vi "Send Write Load Control.vi"(7 "Message Priority (Normal)":T3=enum."Normal", 8 "error in (no error)":errorcluster, 10 "Load_Control":T1, 11 "Message Enqueuer":refnum<class "Message Enqueuer.lvclass">) -> (0 "error out":errorcluster, 3 "Message Enqueuer out":refnum<class "Message Enqueuer.lvclass">)   [LabVIEW 2018, in "Load Actor.lvlib" / "Write Load Control Msg.lvclass"]
doc: "This VI sends the message to an actor."
uses:
  Write Load Control Msg.lvclass
  <vilib>/ActorFramework/Message Enqueuer/Message Enqueuer.lvclass
  <vilib>/ActorFramework/Message Enqueuer/Message Priority.ctl
  <vilib>/ORNL/CSEISMIC DDS/CSEISMIC DDS Base/Data Types/Load_Control.ctl
  <vilib>/ORNL/CSEISMIC DDS/CSEISMIC DDS Base/Data Types/Controls/DeviceID.ctl
  C:/Program Files (x86)/National Instruments/LabVIEW 2018/vi.lib/ActorFramework/Message/Message.lvclass
  Write Load Control Msg.lvclass/Write Load Control Msg.ctl
  <vilib>/ActorFramework/Message Enqueuer/Message Enqueuer.lvclass/Message Enqueuer.ctl
  <vilib>/ActorFramework/Message Priority Queue/Priority Enqueue.vi
  <vilib>/ORNL/CSEISMIC DDS/CSEISMIC DDS Base/CSEISMIC DDS.lvclass
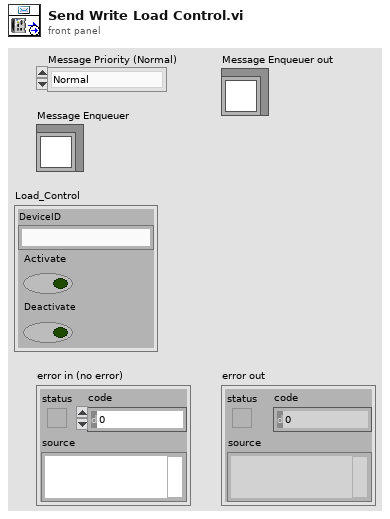
[diagram p1: front panel]
types:
  T1 = typedef "CSEISMIC DDS.lvlib/CSEISMIC DDS.lvclass/Load_Control.ctl" = cluster{"DeviceID":T2, "Activate":bool, "Deactivate":bool}
  T2 = typedef "CSEISMIC DDS.lvlib/CSEISMIC DDS.lvclass/DeviceID.ctl" = string
  T3 = typedef "Actor Framework.lvlib/Message Enqueuer.lvclass/Message Priority.ctl" = enum16{"Low", "Normal", "High"}
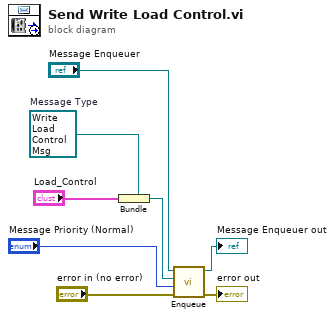
[diagram p0: block diagram]
diagram:
  w5 = refnum<class "Write Load Control Msg.lvclass"> refnum  # Message Type
  n1 = Bundle(cluster=w5, "Load_Control") -> (w4:refnum<class "Write Load Control Msg.lvclass">)
  n2 = call <vilib>:"Enqueue.vi"("error in (no error)"="error in (no error)", "Message Priority (Normal)"="Message Priority (Normal)", "Message"=w4, "Message Enqueuer in"="Message Enqueuer") -> ("error out"=→"error out":errorcluster, "Message Enqueuer out"=→"Message Enqueuer out":refnum<class "Message Enqueuer.lvclass">)  [unwired: 6 in]
